vi "Save Port Settings to JSON.vi"(11 "Port settings":T1={"VISA resource"="", "BAUD"=9600, "Parity"=FALSE, "LDO"=2, "LAI"=3, "Control"=1, "Period"=500}) -> ()   [LabVIEW 2020, in "GUI.lvlib" / "GUI.lvclass"]
uses:
  GUI.lvclass
  Modbus/Modbus/Port Settings.ctl
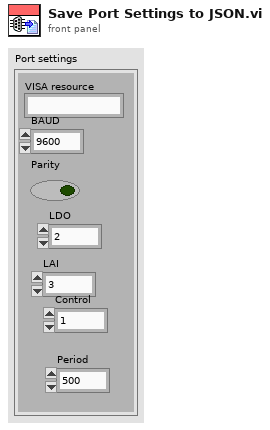
[diagram p1: front panel]
types:
  T1 = typedef "Port Settings.ctl" = cluster{"VISA resource":string, "BAUD":u16, "Parity":bool, "LDO":u16, "LAI":u16, "Control":u16, "Period":u16}
  T2 = enum16{"open", "replace", "create", "open or create", "replace or create", "replace or create with confirmation"}
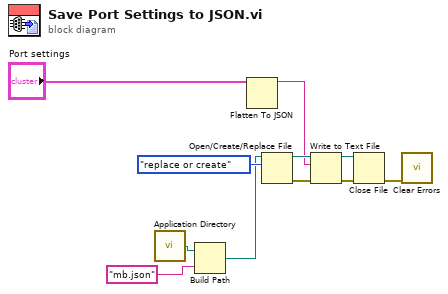
[diagram p0: block diagram]
diagram:
  n1 = call <vilib>:"Application Directory.vi"() -> ("Application Directory"=w9:path)
  n2 = Build Path(base path=w9, name or relative path="mb.json") -> (appended path=w3:path)
  n3 = Flatten To JSON(anything="Port settings") -> (JSON string=w2:string)  [unwired: 2 in, 1 out]
  n4 = Open/Create/Replace File(file path (use dialog)=w3, operation (0:open)=T2."replace or create") -> (refnum out=w6:refnum<file>, error out=w7:errorcluster)  [unwired: 4 in, 1 out]
  n5 = Write to Text File(file (use dialog)=w6, text=w2, error in=w7) -> (refnum out=w4:refnum<file>, error out=w5:errorcluster)  [unwired: 1 in, 1 out]
  n6 = Close File(refnum=w4, error in=w5) -> (error out=w1:errorcluster)  [unwired: 1 out]
  n7 = call <vilib>:"Clear Errors.vi"("error in (no error)"=w1) -> ()  [unwired: 5 in, 2 out]
